vi "Process data.vi"(8 "error in (no error)":errorcluster, 10 "input array":dbl[][](array[numeric]), 11 "ExampleClassDScaffold in":refnum<class "ExampleClassDScaffold.lvclass">) -> (0 "error out":errorcluster, 2 "output array":dbl[][](array[numeric]), 3 "ExampleClassDScaffold out":refnum<class "ExampleClassDScaffold.lvclass">)   [LabVIEW 2012, in "ExampleClassDScaffold.lvclass"]
uses:
  ExampleClassDScaffold.lvclass
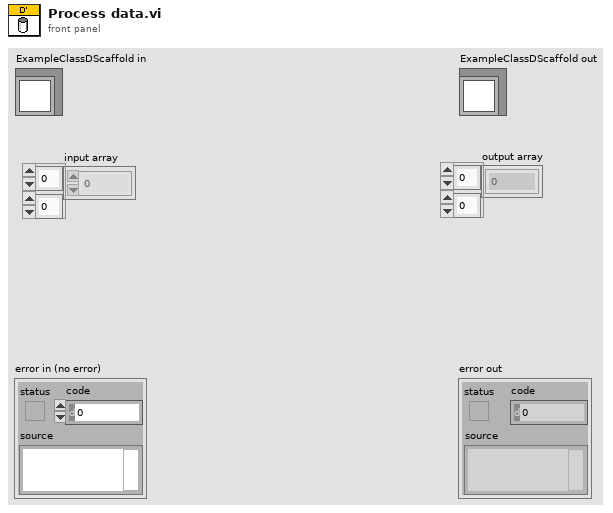
[diagram p1: front panel]
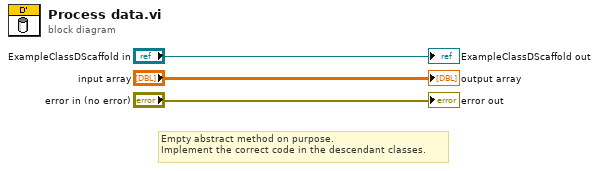
[diagram p0: block diagram]
diagram:
  # "Empty abstract method on purpose.\nImplement the correct code in the descendant classes."
  "error out" <- "error in (no error)"
  "ExampleClassDScaffold out" <- "ExampleClassDScaffold in"
  "output array" <- "input array"
